vi "Install Data Plugin.vi"(0 "reference in":refnum<class "HeadAcousticHDF.lvclass">, 5 "error in (no error)":errorcluster) -> (13 "Successful Install?":bool, 14 "reference out":refnum<class "HeadAcousticHDF.lvclass">, 19 "error out":errorcluster)   [LabVIEW 2020, in "HeadAcousticHDF.lvclass"]
uses:
  HeadAcousticHDF.lvclass
  <vilib>/Platform/storage/utility/Register DataPlugin by URI.vi
  API/Generic Utilities_class/Generic Utilities.lvclass
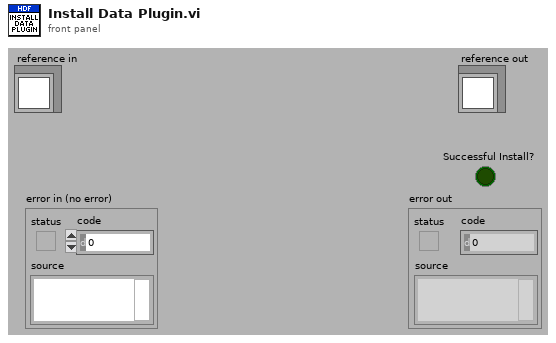
[diagram p1: front panel]
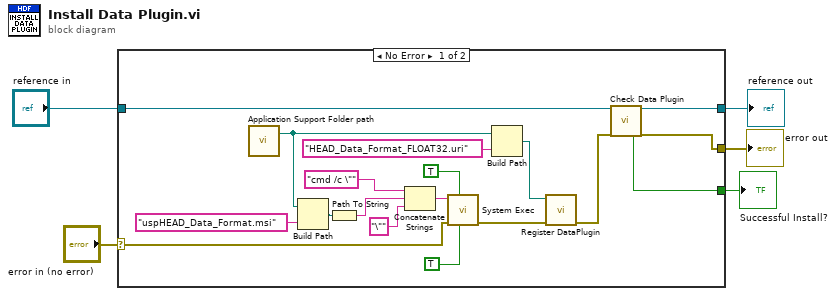
[diagram p0: block diagram]
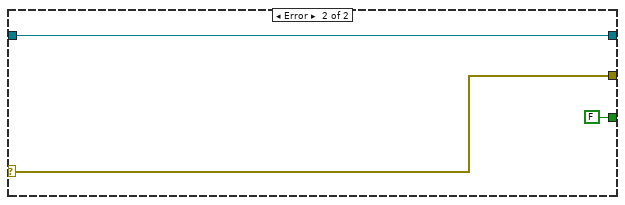
[diagram p2: hidden frame]
diagram:
  n1 = case shown="No Error" "error in (no error)" {
    selector: "error in (no error)" -> [w22 w26]
    tunnel: [w15 w26] -> w4
    tunnel: [w17 w25] -> w2
    tunnel: "reference in" -> [w18 w25]
    tunnel: [w14 FALSE ("HDF Plugin OK?")] -> w1
    frame No Error {
      n2 = call "Application Support Folder path.vi"() -> ("Support path"=w6:path)  [unwired: 19 in]
      n3 = Build Path(base path=w6, name or relative path="uspHEAD_Data_Format.msi") -> (appended path=w12:path)
      n4 = Path To String(path=w12) -> (string=w10:string)
      n5 = Concatenate Strings("cmd /c \"" ("string"), w10, "\"" ("string")) -> (w9:string)
      n6 = call <vilib>:"System Exec.vi"("run minimized? (F)"=TRUE, "wait until completion? (T)"=TRUE, "error in (no error)"=w22, "command line"=w9) -> ("error out"=w21:errorcluster)  [unwired: 4 in, 3 out]
      n7 = Build Path(base path=w6, name or relative path="HEAD_Data_Format_FLOAT32.uri") -> (appended path=w19:path)
      n8 = call-poly <vilib>:"Register DataPlugin.vi"("error in (no error)"=w21, "DataPlugin URI path (*.uri)"=w19) -> ("error out"=w16:errorcluster)  [unwired: 7 in, 2 out]
      n9 = call "Check Data Plugin.vi"("reference in"=w18, "error in (no error)"=w16) -> ("HDF Plugin OK?"=w14:bool, "reference out"=w17:refnum<class "HeadAcousticHDF.lvclass">, "error out"=w15:errorcluster)  [unwired: 15 in]
    }
    frame Error {
    }
  }
  "error out" <- w4
  "reference out" <- w2
  "Successful Install?" <- w1
